vi "Write dest_endpoint.vi"(8 "error in (no error)":errorcluster, 10 "dest_endpoint":string, 11 "Zigbee_Send_Msg in":refnum<class "Zigbee_Send_Msg.lvclass">) -> (0 "error out":errorcluster, 3 "Zigbee_Send_Msg out":refnum<class "Zigbee_Send_Msg.lvclass">)   [LabVIEW 2020, in "Library Test.lvlib" / "Zigbee_Send_Msg.lvclass"]
uses:
  Zigbee_Send_Msg.lvclass
  Zigbee_Send_Msg.lvclass/Zigbee_Send_Msg.ctl
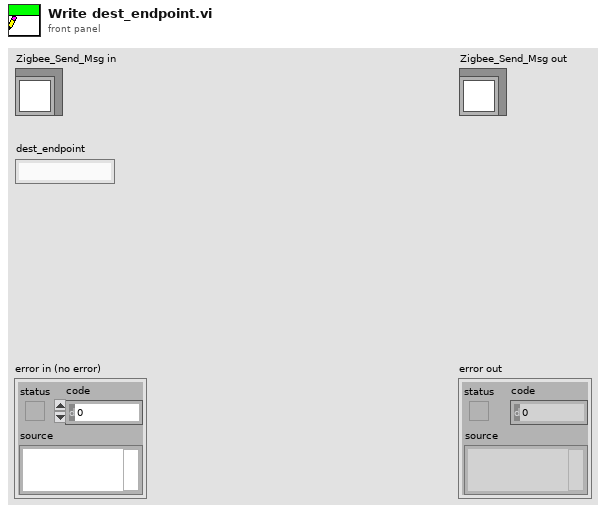
[diagram p1: front panel]
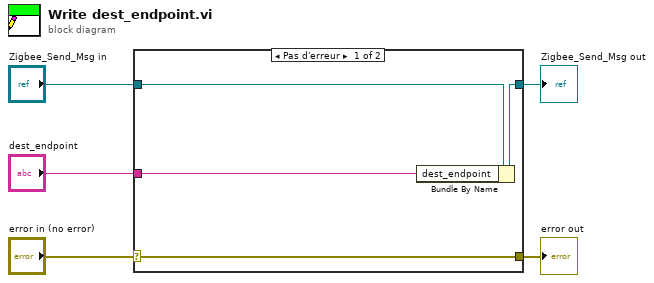
[diagram p0: block diagram]
diagram:
  n1 = case shown="Pas d'erreur" "error in (no error)" {
    selector: "error in (no error)" -> [w9 w10]
    tunnel: [w9 w10] -> w4
    tunnel: [w7 w11] -> w2
    tunnel: "Zigbee_Send_Msg in" -> [w8 w11]
    tunnel: "dest_endpoint" -> [w6 _]
    frame No Error {
      n2 = Bundle By Name(cluster=w8, "dest_endpoint"=w6) -> (w7:refnum<class "Zigbee_Send_Msg.lvclass">)
    }
    frame Error {
    }
  }
  "error out" <- w4
  "Zigbee_Send_Msg out" <- w2
